vi "FTW-Endpoint-CreateReader.vi"(0 "FTW-Endpoint In":refnum<class "FTW-Endpoint.lvclass">, 5 "Address":string, 9 "Timeout":i32=1000 format="%dmsec", 11 "error in":errorcluster) -> (4 "FTW-Endpoint Out":refnum<class "FTW-Endpoint.lvclass">, 6 "Actual Address":string, 15 "error out":errorcluster)   [LabVIEW 2013, in "FTW-Endpoint.lvclass"]
uses:
  FTW-Endpoint.lvclass
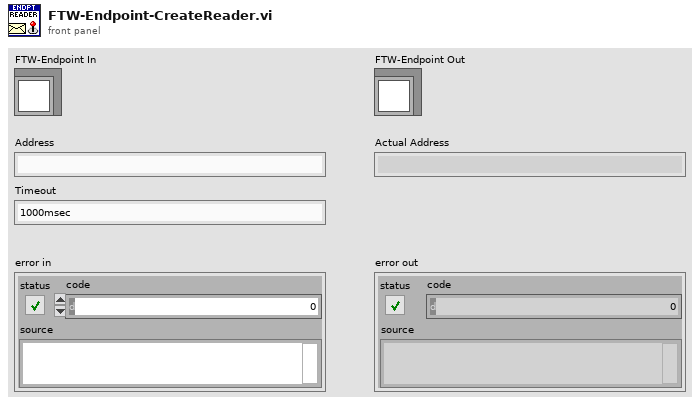
[diagram p1: front panel]
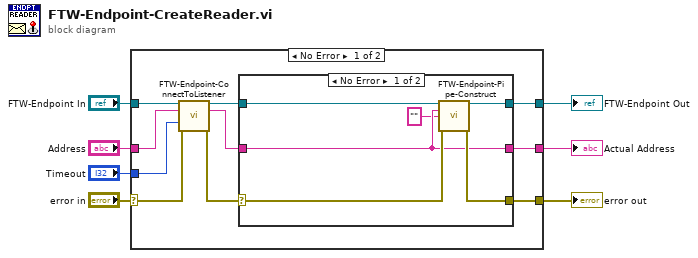
[diagram p0: block diagram]
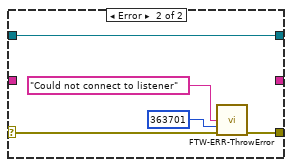
[diagram p2: hidden frame]
diagram:
  n1 = case shown="No Error" "error in" {
    selector: "error in" -> [w14 w30]
    tunnel: [w17 w30] -> w7
    tunnel: [w16 w29] -> w6
    tunnel: "FTW-Endpoint In" -> [w12 w29]
    tunnel: "Address" -> [w10 _]
    tunnel: [w15 _] -> w2
    tunnel: "Timeout" -> [w8 _]
    frame No Error {
      n2 = call-dynamic "FTW-Endpoint-ConnectToListener.vi"("FTW-Endpoint In"=w12, "Address"=w10, "Timeout"=w8, "error in"=w14) -> ("FTW-Endpoint Out"=w11:refnum<class "FTW-Endpoint.lvclass">, "Actual Address"=w9:string, "error out"=w13:errorcluster)  [unwired: 9 in]
      n3 = case shown="No Error" w13 {
        selector: w13 -> [w23 w27]
        tunnel: w11 -> [w21 w28]
        tunnel: [w22 w26] -> w17
        tunnel: [w20 w28] -> w16
        tunnel: w9 -> [w19 _]
        tunnel: [w19 _] -> w15
        frame No Error {
          n4 = call-dynamic "FTW-Endpoint-Pipe-Construct.vi"("FTW Endpoint"=w21, "Address"=w19, "Requested Identity"="", "error in"=w23) -> ("FTW Endpoint out"=w20:refnum<class "FTW-Endpoint.lvclass">, "error out"=w22:errorcluster)  [unwired: 9 in, 1 out]
        }
        frame Error {
          n5 = call "FTW-ERR-ThrowError.vi"("Error Message"="Could not connect to listener", "Error Code"=363701, "error in"=w27) -> ("error out"=w26:errorcluster)  [unwired: 12 in]
        }
      }
    }
    frame Error {
    }
  }
  "FTW-Endpoint Out" <- w6
  "error out" <- w7
  "Actual Address" <- w2
